vi "GetCtrlRefByNameGen.vi"(7 "Commandes []":refnum<vi>[](array[refnum]), 8 "ErrorIn(No Error)":errorcluster caption="entrée d'erreur (pas d'erreur)", 9 "ControlName":string, 10 "InclTabCTrl":bool, 11 "VIRef":refnum<vi>) -> (0 "sortie d'erreur":errorcluster, 2 "ControlsRefs":refnum<vi>, 3 "ControlsNames":string[](array[string]))   [LabVIEW 2019]
uses:
  Programmes Labview/LabscanV1A/DevicesClass/InstrumentsClass/DAQ6363/DAQ6363.lvclass
  <vilib>/Utility/error.llb/Error Cluster From Error Code.vi
  <vilib>/ErrorRing/Error Ring.xnode
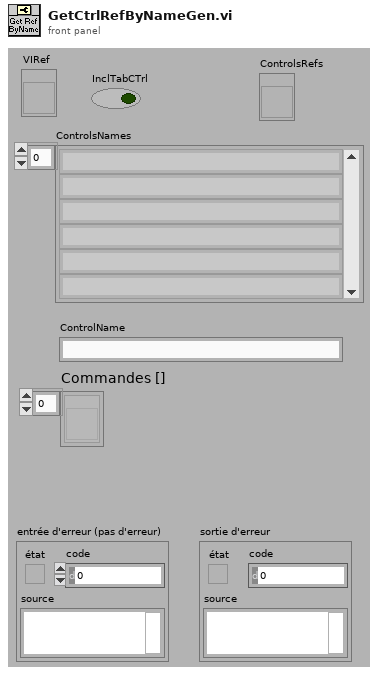
[diagram p1: front panel]
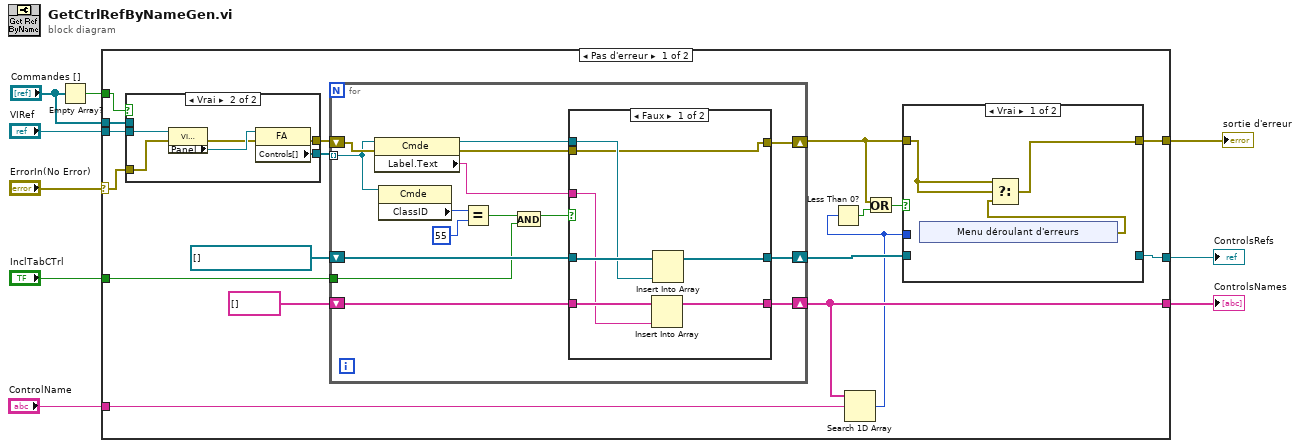
[diagram p0: block diagram]
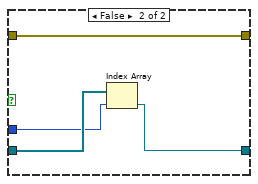
[diagram p3: hidden frame]
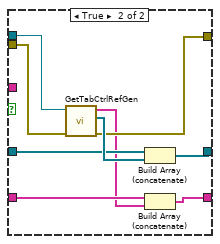
[diagram p4: hidden frame]
diagram:
  n1 = Empty Array?(array="Commandes []") -> (empty?=w2:bool)
  n2 = case shown="Pas d'erreur" "ErrorIn(No Error)" {
    selector: "ErrorIn(No Error)" -> [w25 w79]
    tunnel: [w18 w79] -> w8
    tunnel: "VIRef" -> [w27 _]
    tunnel: [w20 _] -> w6
    tunnel: "InclTabCTrl" -> [w23 _]
    tunnel: "ControlName" -> [w19 _]
    tunnel: [w16 _] -> w3
    tunnel: w2 -> [w10 _]
    tunnel: "Commandes []" -> [w11 _]
    frame No Error {
      n3 = case shown="Vrai" w10 {
        tunnel: w27 -> [_ w33]
        tunnel: [w29 w32] -> w26
        tunnel: w25 -> [w28 w30]
        tunnel: [w28 w31] -> w24
        tunnel: w11 -> [w29 _]
        frame False {
        }
        frame True {
          n4 = property class="VI (strict)"(reference=w33, error in=w30) -> (error out=w34:errorcluster, "Panel"=w35:refnum<vi>)  [unwired: 1 out]
          n5 = property class="FA"(reference=w35, error in=w34) -> (error out=w31:errorcluster, "Controls[]"=w32:refnum<vi>[])  [unwired: 1 out]
        }
      }
      n6 = for {
        tunnel: w26 -> [w61] mode=indexing
        shift-right: [w50] -> w13
        shift-left: w24 -> [w62]
        shift-right: [w55] -> w17
        shift-left: refnum<vi>[] [] -> [w54]
        shift-right: [w53] -> w20
        shift-left: string[] [] -> [w51]
        tunnel: w23 -> [w49]
        n7 = property class="Cmde"(reference=w61, error in=w62) -> (reference out=w57:refnum<vi>, error out=w52:errorcluster, "Label.Text"=w58:string)
        n8 = property class="Cmde"(reference=w61) -> ("ClassID"=w60:u32)  [unwired: 1 in, 2 out]
        n9 = Equal?(x=w60, y=u32 55) -> (x = y?=w56:bool)
        n10 = And(x=w56, y=w49) -> (x .and. y?=w48:bool)
        n11 = case shown="Faux" w48 {
          tunnel: w58 -> [w65 _]
          tunnel: w57 -> [w64 w78]
          tunnel: [w69 w75] -> w55
          tunnel: w54 -> [w68 w73]
          tunnel: [w67 w76] -> w53
          tunnel: w52 -> [w63 w72]
          tunnel: w51 -> [w66 w77]
          tunnel: [w63 w71] -> w50
          frame False {
            n12 = Insert Into Array(array=w66, new element=w65) -> (w67:string[])  [unwired: 1 in]
            n13 = Insert Into Array(array=w68, new element=w64) -> (w69:refnum<vi>[])  [unwired: 1 in]
          }
          frame True {
            n14 = call <userlib>:"GetTabCtrlRefGen.vi"("ErrorIn(No Error)"=w72, "CommandRef"=w78) -> ("sortie d'erreur"=w71:errorcluster, "ControlsRefs"=w74:refnum<vi>[], "ControlsNames"=w70:string[])  [unwired: 7 in]
            n15 = Build Array (concatenate)(w73, w74) -> (w75:refnum<vi>[])
            n16 = Build Array (concatenate)(w77, w70) -> (w76:string[])
          }
        }
      }
      n17 = Search 1D Array(1D array=w20, element=w19) -> (index of element=w12:i32)  [unwired: 1 in]
      n18 = Less Than 0?(x=w12) -> (x < 0?=w14:bool)
      n19 = Or(x=w13, y=w14) -> (x .or. y?=w15:bool)
      n20 = case shown="Vrai" w15 {
        tunnel: [w37 w47] -> w18
        tunnel: w13 -> [w38 w47]
        tunnel: w17 -> [_ w46]
        tunnel: [_ w45] -> w16
        tunnel: w12 -> [_ w44]
        frame True {
          n21 = xnode "Menu déroulant d'erreurs"() -> ("sortie d'erreur"=w36:errorcluster)
          n22 = Select(t=w38, s=w38, f=w36) -> (s? t:f=w37:errorcluster)
        }
        frame False {
          n23 = Index Array(array=w46, index=w44) -> (element=w45:refnum<vi>)
        }
      }
    }
    frame Error {
    }
  }
  "sortie d'erreur" <- w8
  "ControlsNames" <- w6
  "ControlsRefs" <- w3
